vi "Init.vi"(8 "error in (no error)":errorcluster, 10 "Connection String":string, 11 "CameraSim in":refnum<class "CameraI2COUSB.lvclass">) -> (0 "error out":errorcluster, 3 "CameraSim out":refnum<class "CameraI2COUSB.lvclass">)   [LabVIEW 2020, in "Camera.lvlib" / "CameraI2COUSB.lvclass"]
doc: "Inizialize camera object\n\n<b> ConnectionString:</b> String with parameters needed to connecting to camera. The parameters are separate by ::\nThe format is: <Vid>::<Pid>::<Device Index>::<Clock Rate>::<Provider Name>"
uses:
  CameraI2COUSB.lvclass
  I2CDriver/II2COUSB/II2COUSB/ConnectionParams.ctl
  I2CDriver/II2COUSB/II2COUSB/II2COUSB.lvclass
  CameraI2COUSB.lvclass/CameraI2COUSB.ctl
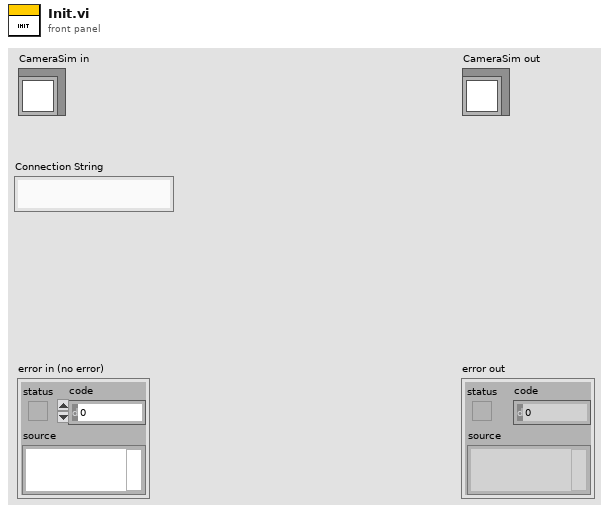
[diagram p1: front panel]
types:
  T1 = typedef "II2COUSB.lvlib/II2COUSB.lvclass/ConnectionParams.ctl" = cluster{"Vid":u16, "Pid":u16, "Device Index":u32, "u32_I2Cclk":u32}
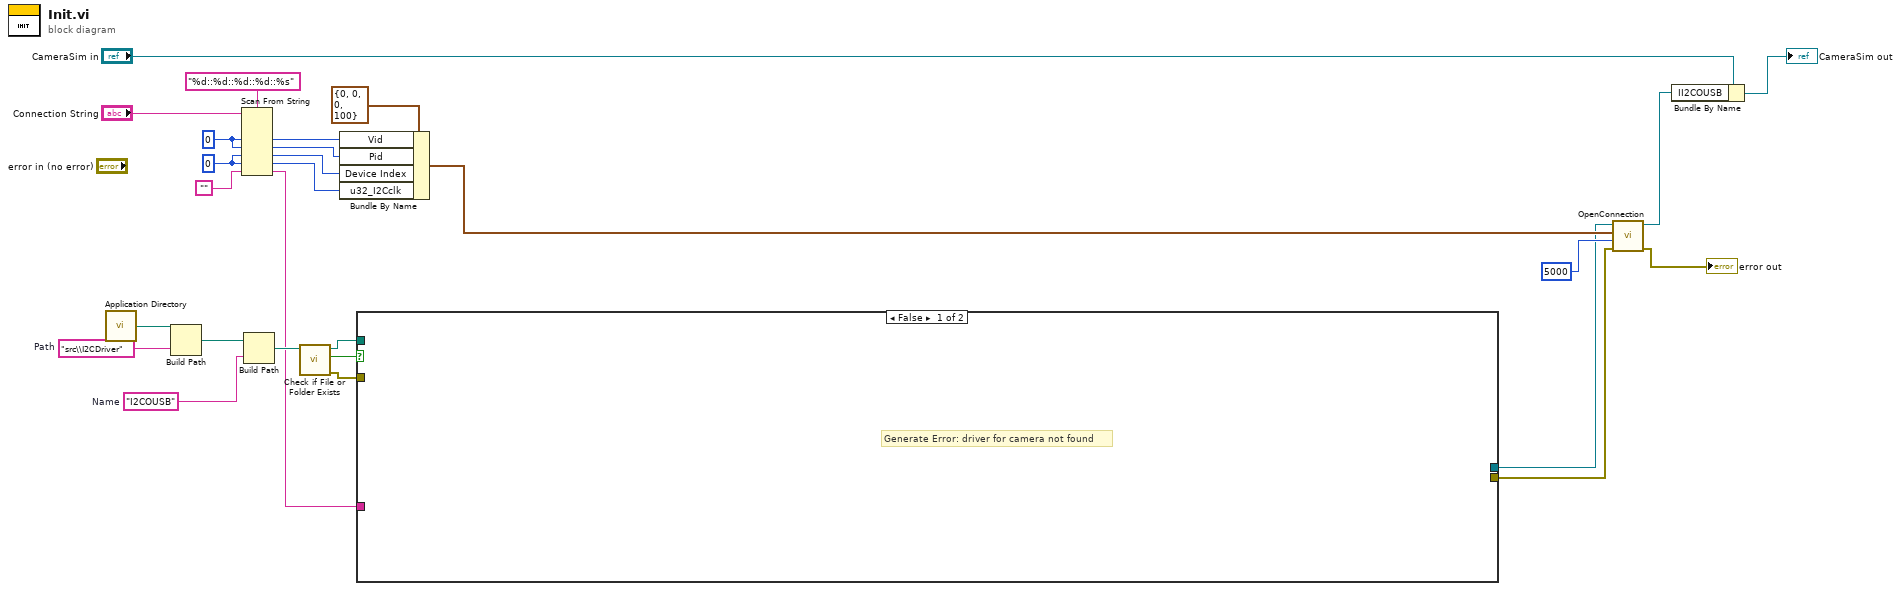
[diagram p0: block diagram]
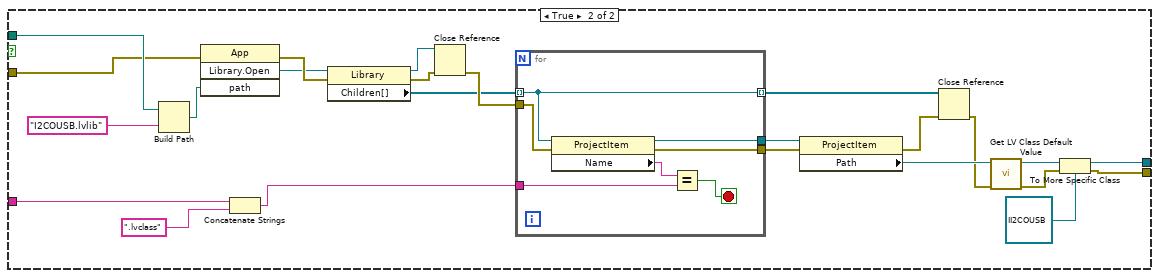
[diagram p2: hidden frame]
diagram:
  w17 = u32 0
  w18 = u16 0
  w24 = "I2COUSB"  # Name
  w26 = "src\\I2CDriver"  # Path
  n1 = call <vilib>:"Application Directory.vi"() -> ("Application Directory"=w27:path)
  n2 = Build Path(base path=w27, name or relative path=w26) -> (appended path=w25:path)
  n3 = Scan From String(format string="%d::%d::%d::%d::%s", input string="Connection String", default 1=w18, default 2=w18, default 3=w17, default 4=w17, default 5="") -> (output 1=w14:u16, output 2=w13:u16, output 3=w12:u32, output 4=w11:u32, output 5=w2:string)  [unwired: 2 in, 3 out]
  n4 = Build Path(base path=w25, name or relative path=w24) -> (appended path=w23:path)
  n5 = call <vilib>:"Check if File or Folder Exists.vi"("path"=w23) -> ("error out"=w20:errorcluster, "file or folder exists?"=w22:bool, "dup path"=w21:path)  [unwired: 8 in]
  n6 = Bundle By Name(cluster=T1 {"Vid"=0, "Pid"=0, "Device Index"=0, "u32_I2Cclk"=100} ("Connection Params"), "Vid"=w14, "Pid"=w13, "Device Index"=w12, "u32_I2Cclk"=w11) -> (w10:T1)
  n7 = case shown="False" w22 {
    tunnel: w21 -> [_ w49]
    tunnel: w20 -> [_ w38]
    tunnel: [_ w32] -> w8
    tunnel: [_ w31] -> w7
    tunnel: w2 -> [_ w30]
    frame False {
      # "Generate Error: driver for camera not found"
    }
    frame True {
      n8 = Build Path(base path=w49, name or relative path="I2COUSB.lvlib") -> (appended path=w47:path)
      n9 = invoke class="App" method="Library.Open"(error in=w38, "path"=w47) -> (error out=w51:errorcluster, "Open Library"=w50:refnum<vi>)  [unwired: 2 in, 2 out]
      n10 = Concatenate Strings(w30, ".lvclass" ("y")) -> (w28:string)
      n11 = property class="Library"(reference=w50, error in=w51) -> (reference out=w45:refnum<vi>, error out=w46:errorcluster, "Children[]"=w41:refnum<vi>[])
      n12 = Close Reference(reference=w45, error in (no error)=w46) -> (error out=w44:errorcluster)
      n13 = for {
        tunnel: w41 -> [w53] mode=indexing
        tunnel: w44 -> [w57]
        tunnel: [w55] -> w43
        tunnel: [w54] -> w42
        tunnel: [w53] -> w39 mode=indexing
        tunnel: w28 -> [w52]
        stop <- w56 stop-if-true
        n14 = property class="ProjectItem"(reference=w53, error in=w57) -> (reference out=w55:refnum<vi>, error out=w54:errorcluster, "Name"=w58:string)
        n15 = Equal?(x=w58, y=w52) -> (x = y?=w56:bool)
      }
      n16 = property class="ProjectItem"(reference=w43, error in=w42) -> (error out=w40:errorcluster, "Path"=w37:path)  [unwired: 1 out]
      n17 = Close Reference(reference=w39, error in (no error)=w40) -> (error out=w36:errorcluster)
      n18 = call <vilib>:"Get LV Class Default Value.vi"("error in (no error)"=w36, "class path"=w37) -> ("error out"=w35:errorcluster, "object"=w34:refnum<class>)  [unwired: 8 in]
      n19 = To More Specific Class(target class=refnum<class "II2COUSB.lvclass"> refnum ("II2COUSB.lvlib:II2COUSB.lvclass"), reference=w34, error in=w35) -> (specific class reference=w32:refnum<class "II2COUSB.lvclass">, error out=w31:errorcluster)
    }
  }
  n20 = call-dynamic "OpenConnection.vi"("error in (no error)"=w7, "Timeout (ms)"=u32 5000, "Connection Params"=w10, "II2COUSB in"=w8) -> ("error out"=→"error out":errorcluster, "II2COUSB out"=w3:refnum<class "II2COUSB.lvclass">)  [unwired: 6 in]
  n21 = Bundle By Name(cluster="CameraSim in", "II2COUSB"=w3) -> (→"CameraSim out":refnum<class "CameraI2COUSB.lvclass">)
